vi "4bmilo_jo.vi"() -> ()   [LabVIEW 2010]
uses:
  <vilib>/measure/NI_MABase.lvlib
panel:
  out "Ugen=f(t)":waveform(dbl)(graph)
  out "fgen(Hz)":dbl=10.0 format="%0.2p"
  in  "fmax(Hz)":i32
  in  "krok":i32
  in  "fmin(Hz)":i32
  in  "Typ signálu":T1(ring)
  in  "Ugen(V)":dbl=1.0 format="%0.2p"
  # "Automatizovaný snímač přenosových charakteristik"
  # "Rozmítaný generátor"
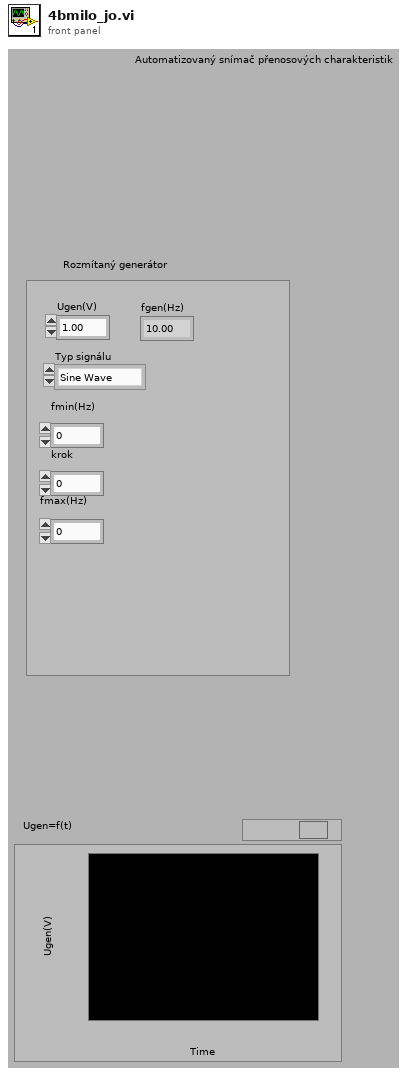
[diagram p1: front panel]
types:
  T1 = enum16{"Sine Wave", "Triangle Wave", "Square Wave", "Sawtooth Wave"}
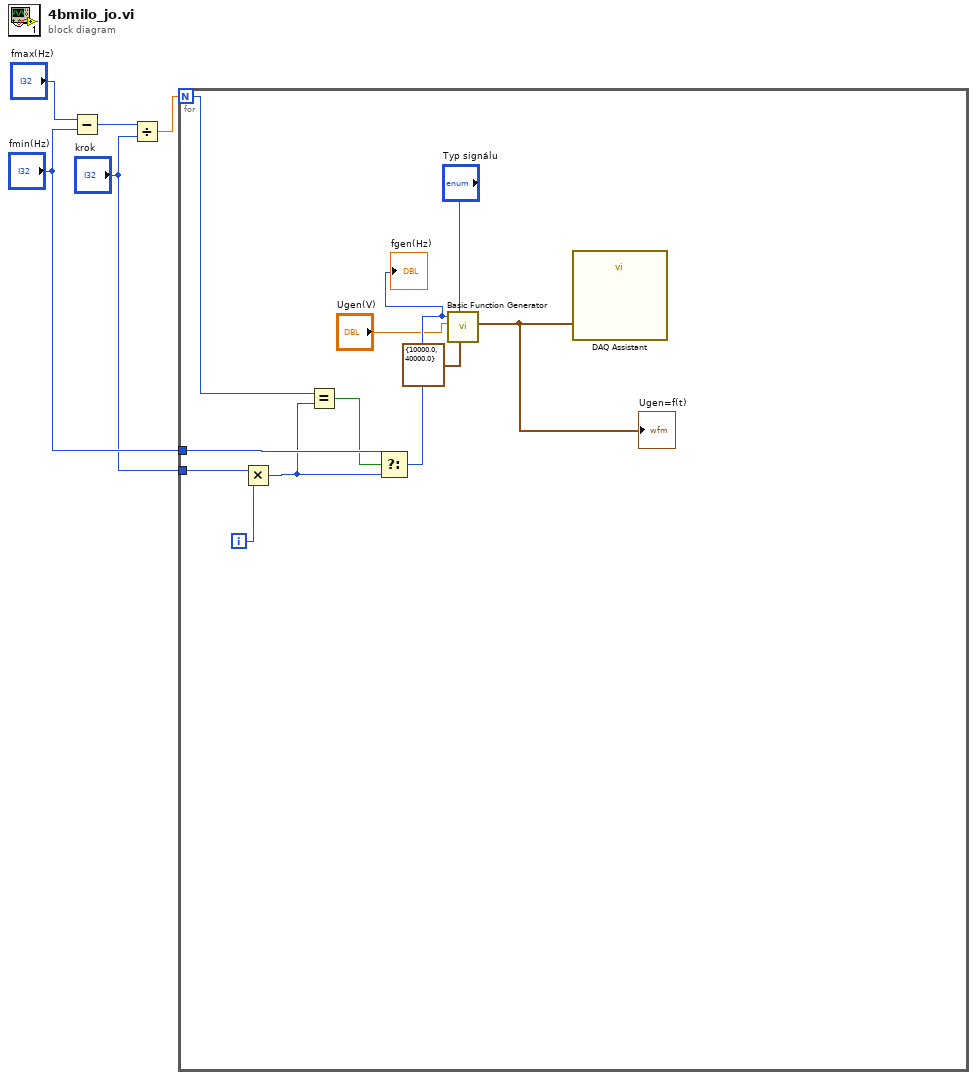
[diagram p0: block diagram]
diagram:
  n1 = Subtract(x="fmax(Hz)", y="fmin(Hz)") -> (x-y=w4:i32)
  n2 = Divide(x=w4, y="krok") -> (x/y=w3:dbl)
  n3 = for {
    N: w3 -> [w11]
    tunnel: "fmin(Hz)" -> [w13]
    tunnel: "krok" -> [w15]
    i -> [w14]
    n4 = Multiply(x=w15, y=w14) -> (x*y=w12:i32)
    n5 = Equal?(x=w11, y=w12) -> (x = y?=w10:bool)
    n6 = Select(t=w13, s=w10, f=w12) -> (s? t:f=w9:i32)
    "fgen(Hz)" <- w9
    n7 = call <vilib>:"Basic Function Generator.vi"("sampling info"=cluster{"Fs":dbl, "#s":dbl} {"Fs"=10000.0, "#s"=40000.0}, "signal type"="Typ signálu", "amplitude"="Ugen(V)", "frequency"=w9) -> ("signal out"=w7:waveform(dbl))  [unwired: 5 in, 2 out]
    "Ugen=f(t)" <- w7
    n8 = call "DAQ Assistant"("data"=w7) -> ()  [unwired: 17 in, 2 out]
  }
